vi "Streamer.vi"(8 "#s":i32=96, 9 "channel number":i32, 10 "stop notifier":refnum<notifier>, 11 "gRPCid in":T1) -> ()   [LabVIEW 2019, in "Signal Provider.lvclass"]
uses:
  Signal Provider.lvclass
  <vilib>/gRPC/LabVIEW gRPC Library/Server API/typeDefs/grpcId.ctl
  <vilib>/Platform/TimedLoop/XDataNode/timing_clust.ctl
  <vilib>/Platform/TimedLoop/XDataNode/nitl_modes.ctl
  <vilib>/Platform/TimedLoop/XDataNode/wakeup.ctl
  Servers/Streamer_server/Streamer_server Class/RPC Messages/Waveform/Waveform_Data.ctl
  <vilib>/platform/TimedLoop/XDataNode/XDataNode.xnode
  <vilib>/Platform/TimedLoop/XDataNode/XDNodeRunTimeDep.lvlib
  Servers/Streamer_server/Streamer_server Class/Streamer_server.lvclass
  <vilib>/gRPC/LabVIEW gRPC Library/gprc-lvsupport-release.lvlib
panel:
  in  "manual stop":bool
  out "data":waveform(dbl)(graph)
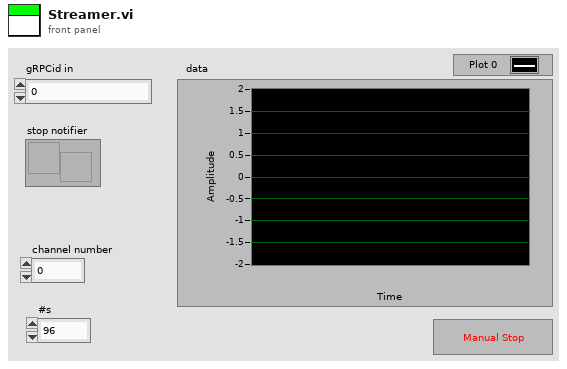
[diagram p1: front panel]
types:
  T1 = typedef "gprc-lvsupport-release.lvlib/grpcId.ctl" = u64
  T2 = typedef "XDNodeRunTimeDep.lvlib/timing_clust.ctl" = cluster{"Expected End [f-1]":u64, "Actual End [f-1]":u64, "Finished Late? [f-1]":bool, "Expected End [i-1]":u64, "Actual End [i-1]":u64, "Finished Late? [i-1]":bool, "Expected Start [i]":u64, "Actual Start [i]":u64, "Expected Start [f]":u64, "Actual Start [f]":u64, "Source Name":string, "Structure Name":string, "Period":i64, "Deadline":i64, "Offset":i64, "Start":i64, "Priority":i32, "Timeout":i32, "Mode":T3, "Wakeup Reason":T4, "Error":errorcluster, "Source Type":string, "Secondary Source Type":string, "Global End Time":u64, "Global Start Time":u64, "Frame Duration":u64, "Iteration Duration":u64, "Assigned CPU":i32, "I/O Scan Engine Mode":u32}
  T3 = typedef "XDNodeRunTimeDep.lvlib/nitl_modes.ctl" = enum32{"No Change", "Process missed periods, maintain original phase", "Discard missed periods, maintain original phase", "Process missed periods, ignore original phase", "Discard missed periods, ignore original phase"}
  T4 = typedef "XDNodeRunTimeDep.lvlib/wakeup.ctl" = enum32{"Normal", "Aborted", "Asynchronous wakeup", "Timing source error", "Timed loop error", "Timeout"}
  T5 = typedef "Streamer_server.lvlib/Streamer_server.lvclass/Waveform_Data.ctl" = cluster{"startTime":dbl, "dt":dbl, "samples":dbl[]}
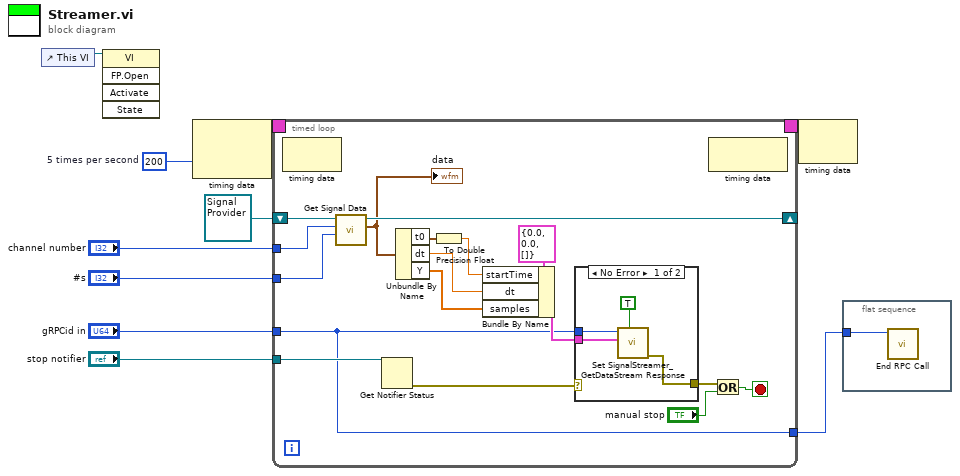
[diagram p0: block diagram]
diagram:
  w8 = i64 200  # 5 times per second
  n1 = control-ref of="This VI"() -> (w3:refnum<vi>)
  n2 = invoke class="VI" method="FP.Open"(reference=w3) -> ()  [unwired: 4 in, 5 out]
  n3 = node-c288(w8) -> (w10:T2)  [unwired: 1 in]
  n4 = timed-loop {
    timing: w10 -> [_]
    timing-out: [_] -> w9
    shift-right: [w26] -> _
    shift-left: refnum<class "Signal Provider.lvclass"> refnum ("Signal Provider.lvclass") -> [w27]
    tunnel: "channel number" -> [w25]
    tunnel: "stop notifier" -> [w24]
    tunnel: "gRPCid in" -> [w11]
    tunnel: "#s" -> [w15]
    tunnel: [w11] -> w1
    stop <- w12 stop-if-true
    n5 = node-c288() -> ()  [unwired: 1 in, 1 out]
    n6 = call "Get Signal Data.vi"("#s"=w15, "channel number"=w25, "Signal Provider in"=w27) -> ("data"=w16:waveform(dbl), "Signal Provider out"=w26:refnum<class "Signal Provider.lvclass">)  [unwired: 6 in, 1 out]
    "data" <- w16
    n7 = Get Notifier Status(notifier=w24) -> (error out=w17:errorcluster)  [unwired: 1 in, 4 out]
    n8 = Unbundle By Name(w16) -> ("t0"=w20:timestamp, "dt"=w19:dbl, "Y"=w18:dbl[])
    n9 = To Double Precision Float(number=w20) -> (double precision float=w21:dbl)
    n10 = Bundle By Name(cluster=T5 {"startTime"=0.0, "dt"=0.0, "samples"=[]} ("Message Data"), "startTime"=w21, "dt"=w19, "samples"=w18) -> (w22:T5)
    n11 = case shown="No Error" w17 {
      selector: w17 -> [_ w32]
      tunnel: w11 -> [w28 _]
      tunnel: w22 -> [w31 _]
      tunnel: [w29 w32] -> w14
      frame No Error {
        n12 = call "Set SignalStreamer_GetDataStream Response.vi"("Streeming? (F)"=TRUE, "Message Data"=w31, "gRPCid in"=w28) -> ("error out"=w29:errorcluster)  [unwired: 8 in]
      }
      frame Error {
      }
    }
    n13 = node-c288() -> ()  [unwired: 1 in, 1 out]
    n14 = Or(x=w14, y="manual stop") -> (x .or. y?=w12:bool)
  }
  n15 = node-c288(w9) -> ()  [unwired: 1 out]
  n16 = flat-sequence {
    tunnel: w1 -> [w35]
    frame #0 {
      n17 = call "End RPC Call.vi"("gRPCid"=w35) -> ()  [unwired: 10 in, 1 out]
    }
  }
